vi "叶绿素a_获取温度和叶绿素值.vi"(8 "error in (no error)":errorcluster caption="错误输入（无错误）", 11 "MB session in":refnum<class "MB_Master.lvclass">) -> (0 "error out":errorcluster caption="错误输出", 2 "输出值":cluster{"温度测量值":sgl, "叶绿素测量值":sgl, "错误标志":u16} {"错误标志" items=["NO Error"=0, "刷子没到位"=255]}, 3 "MB session out":refnum<class "MB_Master.lvclass">)   [LabVIEW 2016, in "斯坦道多参数.lvlib"]
uses:
  <vilib>/Plasmionique/MB Master/MB_Master/MB_Master.lvclass
  <vilib>/Plasmionique/MB Master/MB Master.lvlib
  <vilib>/ptbypt/NI_PtbyPt.lvlib
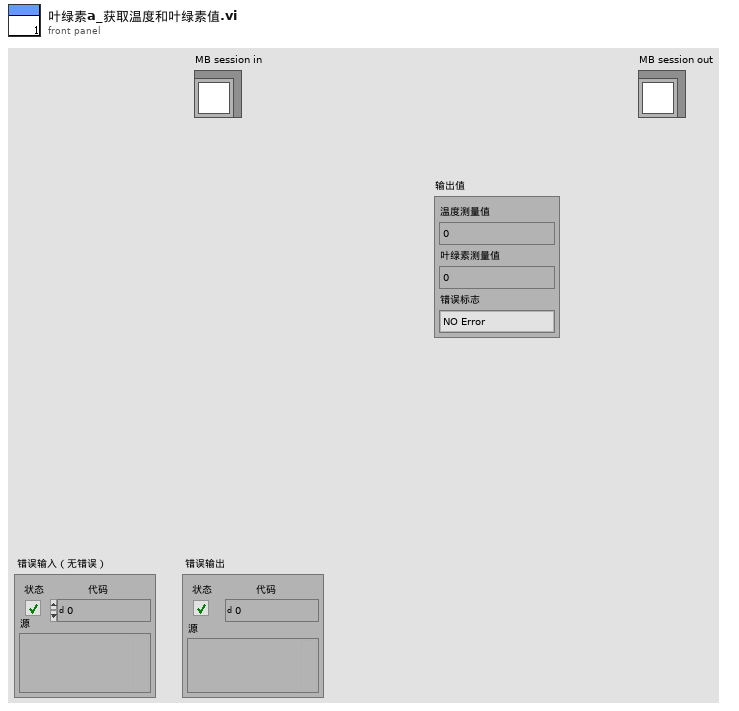
[diagram p1: front panel]
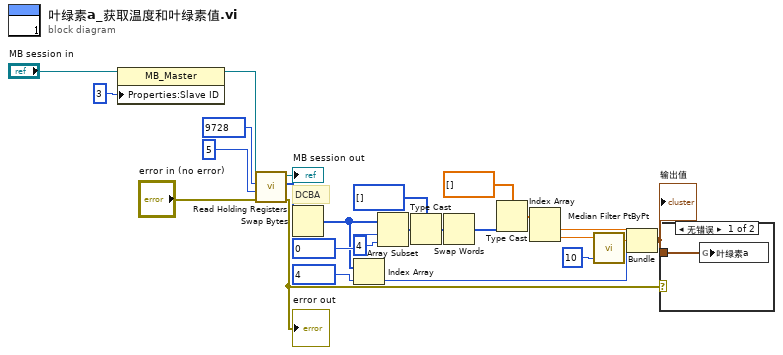
[diagram p0: block diagram]
diagram:
  # "DCBA"
  n1 = property class="MB_Master"(reference="MB session in", "Properties:Slave ID"=u16 3 ("y")) -> (reference out=w14:refnum<class "MB_Master.lvclass">)  [unwired: 1 in, 1 out]
  n2 = call <vilib>:"Read Holding Registers.vi"("error in (no error)"="error in (no error)", "quantity"=u16 5, "starting address"=u16 9728, "MB session in"=w14) -> ("error out"=w7:errorcluster, "Registers"=w10:u16[], "MB session out"=→"MB session out":refnum<class "MB_Master.lvclass">)  [unwired: 5 in]
  "error out" <- w7
  n3 = Swap Bytes(anything=w10) -> (byte swapped=w9:u16[])
  n4 = Index Array(array=w9, index=u16 4 ("starting address")) -> (element=w11:u16)
  n5 = Array Subset(array=w9, index=u16 0 ("starting address"), length=4 ("长度")) -> (w8:u16[])
  n6 = Type Cast(type=u32[] [] ("数组 2"), x=w8) -> (*(type *) &x=w20:u32[])
  n7 = Swap Words(1:w20) -> (0:w22:u32[])
  n8 = Type Cast(type=sgl[] [] ("数组 2"), x=w22) -> (*(type *) &x=w18:sgl[])
  n9 = Index Array(array=w18) -> (element #1=w17:sgl, element #2=w3:sgl)  [unwired: 2 in]
  n10 = call <vilib>:"Median Filter PtByPt.vi"("rank"=10, "x"=w3) -> ("Filtered x"=w2:dbl)  [unwired: 2 in, 1 out]
  n11 = Bundle("数值"=w17, "Filtered x"=w2, w11) -> (w6:cluster{"数值":sgl, "Filtered x":dbl, u16})  [unwired: 1 in]
  "输出值" <- w6
  n12 = case shown="无错误" w7 {
    tunnel: w6 -> [w26 _]
    frame No Error {
      n13 = global write "禹山过程全局变量.vi" "叶绿素a"(w26) -> ()
    }
    frame Error {
    }
  }
